vi "simulation stuff.vi"() -> ()   [LabVIEW 2023]
panel:
  out "XY Graph":cluster{"X":dbl, "Y":dbl}[](graph)
  out "appended array":cluster{dbl, dbl}[](array[cluster])
  out "cluster B":cluster{dbl, dbl}
  out "cluster A":cluster{dbl, dbl}
  in  "angle upper":dbl
  in  "angle lower":dbl
  in  "length upper":dbl
  in  "length lower":dbl
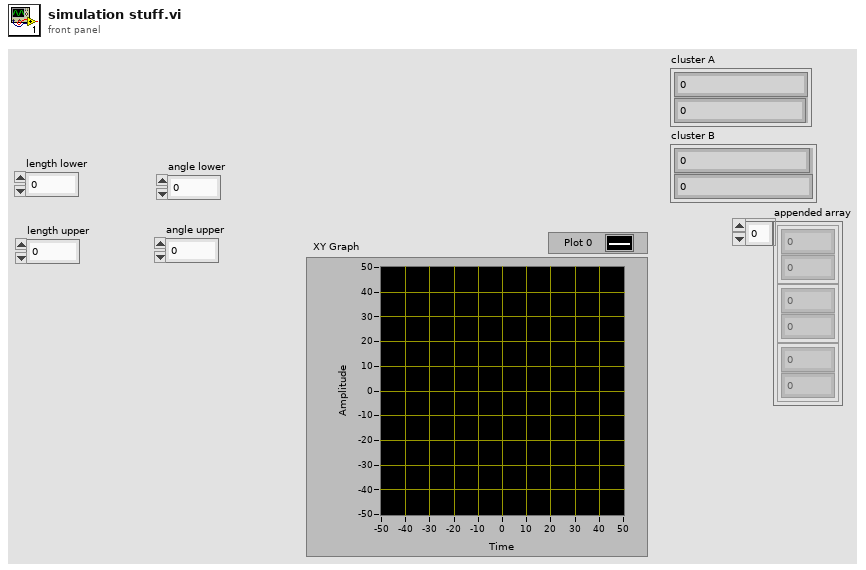
[diagram p1: front panel]
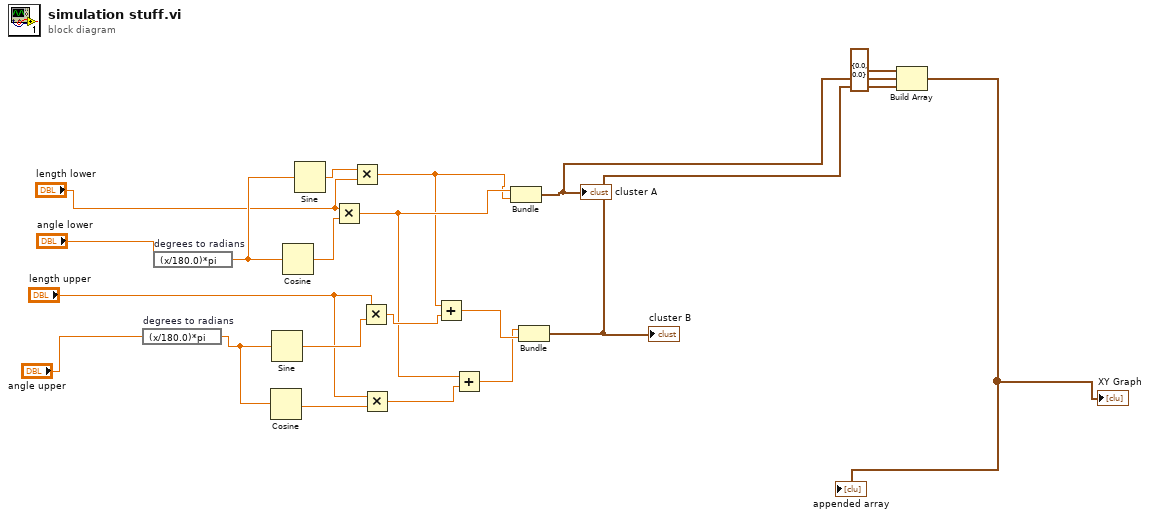
[diagram p0: block diagram]
diagram:
  n1 = expression code="(x/180.0)*pi" "degrees to radians"("angle upper") -> (w17:dbl)
  n2 = expression code="(x/180.0)*pi" "degrees to radians"("angle lower") -> (w19:dbl)
  n3 = Cosine(x=w17) -> (cos(x)=w16:dbl)
  n4 = Sine(x=w17) -> (sin(x)=w13:dbl)
  n5 = Cosine(x=w19) -> (cos(x)=w20:dbl)
  n6 = Sine(x=w19) -> (sin(x)=w18:dbl)
  n7 = Multiply(x="length lower", y=w20) -> (x*y=w4:dbl)
  n8 = Multiply(x=w18, y="length lower") -> (x*y=w3:dbl)
  n9 = Multiply(x="length upper", y=w13) -> (x*y=w14:dbl)
  n10 = Multiply(x="length upper", y=w16) -> (x*y=w15:dbl)
  n11 = Add(x=w3, y=w14) -> (x+y=w6:dbl)
  n12 = Add(x=w4, y=w15) -> (x+y=w5:dbl)
  n13 = Bundle(w4, w3) -> (w12:cluster{dbl, dbl})  [unwired: 1 in]
  "cluster A" <- w12
  n14 = Bundle(w5, w6) -> (w11:cluster{dbl, dbl})  [unwired: 1 in]
  "cluster B" <- w11
  n15 = Build Array(cluster{dbl, dbl} {0.0, 0.0} ("element"), w12, w11) -> (→"appended array" →"XY Graph":cluster{dbl, dbl}[])
